vi "Write State.vi"(8 "error in (no error)":errorcluster, 10 "generator state":T3={"system timing model"=10178, "state"={"RESET"=FALSE, "generator timestamp"=timestamp(0 s since 1904-01-01), "elapsed seconds"=0.0, "elapsed samples"=0, "generation state"=enum."Idle", "time offset at state"=0.0, "samples generated at state"=0, "signal state"=variant}, "duration of state"=0.0, "samples remaining at state"=0} {"system timing model" items=["Finite"=10178, "-"=-1, "Continuous"=10123, "-"=-2, "Settled"=110123, "Averaged"=210123, "Discrete Sweep"=310123, "Continuous Sweep"=410123]}, 11 "signal configuration":refnum<class "SV Signal.lvclass">) -> (0 "error out":errorcluster, 3 "signal configuration":refnum<class "SV Signal.lvclass">)   [LabVIEW 2017, in "SV Signal.lvclass"]
uses:
  <vilib>/addons/_NISVFA/_Generation/Signal Generation/SV Signal/SV Signal.lvclass
  <vilib>/addons/_NISVFA/_Generation/Signal Generation/SV Signal/sv_System Timing Model.ctl
  <vilib>/addons/_NISVFA/_Generation/Signal Generation/SV Signal/sv_Generation State.ctl
  <vilib>/addons/_NISVFA/_Generation/Signal Generation/SV Signal/SV Signal.lvclass/SV Signal.ctl
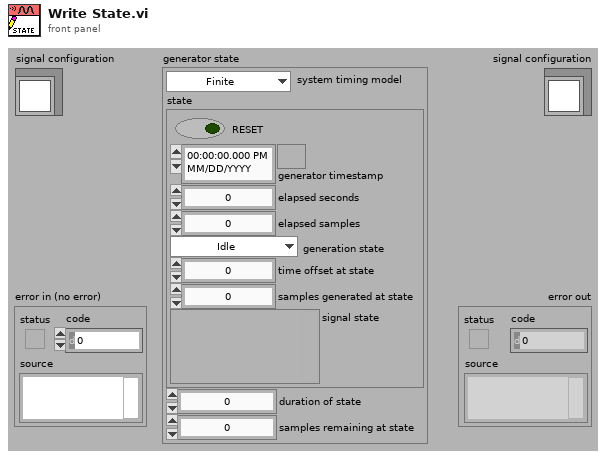
[diagram p1: front panel]
types:
  T1 = typedef "SV Signal.lvclass/sv_System Timing Model.ctl" = i64
  T2 = typedef "SV Signal.lvclass/sv_Generation State.ctl" = enum16{"Idle", "Ramp Up", "Pre-Measurement Settling", "Measurement", "Post-Measurement Settling", "Discrete Sweep Transition", "Ramp Down", "Update"}
  T3 = cluster{"system timing model":T1, "state":cluster{"RESET":bool, "generator timestamp":timestamp, "elapsed seconds":dbl, "elapsed samples":u64, "generation state":T2, "time offset at state":dbl, "samples generated at state":u64, "signal state":variant}, "duration of state":dbl, "samples remaining at state":i32}
  T4 = cluster{"RESET":bool, "generator timestamp":timestamp, "elapsed seconds":dbl, "elapsed samples":u64, "generation state":T2, "time offset at state":dbl, "samples generated at state":u64, "signal state":variant}
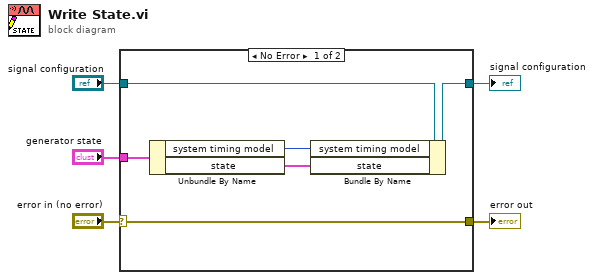
[diagram p0: block diagram]
diagram:
  n1 = case shown="No Error" "error in (no error)" {
    selector: "error in (no error)" -> [w11 w12]
    tunnel: [w11 w12] -> w4
    tunnel: [w9 w13] -> w2
    tunnel: "signal configuration" -> [w10 w13]
    tunnel: "generator state" -> [w8 _]
    frame No Error {
      n2 = Unbundle By Name(w8) -> ("system timing model"=w7:T1, "state"=w6:T4)
      n3 = Bundle By Name(cluster=w10, "system timing model"=w7, "state"=w6) -> (w9:refnum<class "SV Signal.lvclass">)
    }
    frame Error {
    }
  }
  "error out" <- w4
  "signal configuration" <- w2
